vi "Trigger Controls with Data from CAT -sw1.vi"(5 "West ON/Std OFF":bool, 7 "Mode":enum16{"Run", "Hold", "Off"}(ring), 8 "error in":errorcluster, 11 "Com Parms":T2={"VISA resource name"="COM4", "baud rate"=38400, "data bits"=8, "parity"=0, "stop bits"=10, "flow control"=0} {"flow control" items=["None"=0, "XON/XOFF"=1, "RTS/CTS"=2, "DTR/DSR"=4]; "stop bits" items=["1.0"=10, "1.5"=15, "2.0"=20]; "parity" items=["None", "Odd", "Even", "Mark", "Space"]; "data bits" min=5 max=8 step=1}) -> (0 "error out":errorcluster, 3 "Final Output":T3={"Main 1"=TRUE, "Main 2"=TRUE, "Recirc  3"=TRUE, "Scrub 4"=FALSE, "O2 5"=TRUE, "Vent 6"=FALSE, "Boost A 7"=FALSE, "Boost A 8"=TRUE, "Recirc  9"=FALSE, "Scrub 10"=FALSE, "Vent 11"=FALSE, "Boost B 12"=TRUE, "Boost B 13"=TRUE, "Recirc 14"=TRUE, "Scrub 15"=FALSE, "Vent 16"=FALSE, "Main 17"=TRUE, "Boost A 18"=TRUE, "Boost B 19"=TRUE, "Boost F 20"=TRUE, "Vent 2 21"=FALSE})   [LabVIEW 2012]
uses:
  <vilib>/Platform/TimedLoop/XDataNode/XDataNode.xnode
  <vilib>/Platform/TimedLoop/XDataNode/nitl_modes.ctl
  <vilib>/Platform/TimedLoop/XDataNode/XDNodeRunTimeDep.lvlib
  <vilib>/Platform/TimedLoop/XDataNode/wakeup.ctl
  <vilib>/Platform/TimedLoop/XDataNode/timing_clust.ctl
  Type Defs/Final Output.ctl
  Type Defs/CO2 Settings.ctl
  Type Defs/AD Settings.ctl
  Type Defs/Output Values.ctl
  Type Defs/Output Switches.ctl
  Type Defs/Data Reading.ctl
panel:
  out "Time":string="16:44:30"
  out "Date":string="03/29/13"
  in  "Stop Button":bool
  in  "Tab Control":T1(tab)=enum."AD Settings"
  in  "Other Outputs":cluster{"Alarm":bool, "Heater":bool}
  in  "Period":i64=1000
  in  "Set Point Alt":dbl=1600.0 min=0.0 max=10000.0 step=1.0
  out "Cycles":i32=627
  out "CO2 ppm":u32(slide)=465 scale=0.0..10000.0
  out "Alt Dif M":dbl(slide)=-1619.283557610342 scale=-1000.0..1000.0 scale format="%.1f"
  out "AD Output":T3={"Main 1"=TRUE, "Main 2"=TRUE, "Recirc  3"=TRUE, "Scrub 4"=FALSE, "O2 5"=TRUE, "Vent 6"=FALSE, "Boost A 7"=FALSE, "Boost A 8"=TRUE, "Recirc  9"=FALSE, "Scrub 10"=FALSE, "Vent 11"=FALSE, "Boost B 12"=TRUE, "Boost B 13"=TRUE, "Recirc 14"=TRUE, "Scrub 15"=FALSE, "Vent 16"=FALSE, "Main 17"=TRUE, "Boost A 18"=TRUE, "Boost B 19"=TRUE, "Boost F 20"=TRUE, "Vent 2 21"=FALSE}
  out "AD State":T3
  out "Data Read":T4={"Date"="03/29/13", "Time"="16:44:31", "CO2- ppm"=467, "Last Ctrl Word"=5191831, "O2-1 ppm"=210267, "O2-2 ppm"=210262, "Temp MB"=23.23, "Temp Sensor Module"=26.21, "Press mB"=1011.26} {"Last Ctrl Word" format="%.0x"}
  out "Force Output":T5
  out "Force State":T3
  out "Alt Calc":dbl=-19.283557610342072
  in  "CO2 Settings":T6={"Run C1"={"A-1,  1"=inf, "A-3,  2"=inf, "A-4, 3"=9000.0, "A-5, 4"=8800.0, "ABCD-7, 5"=9600.0, "A-8, 6"=9200.0, "B-1,  7"=3400.0, "B-3, 8"=3400.0, "B-4,  9"=9000.0, "B-5, 10"=8800.0, "B-8, 11"=9200.0, "C-1, 12"=1800.0, "C-3, 13"=1800.0, "C-4, 14"=9000.0, "C-5,  15"=8800.0, "C-8, 16"=9200.0, "D-1, 17"=inf, "D-3, 18"=3400.0, "D-4,  19"=1800.0, "D-5,  20"=7000.0, "D-8,  21"=9200.0}, "Run C2"={"A-1,  1"=inf, "A-3,  2"=inf, "A-4, 3"=8800.0, "A-5, 4"=8600.0, "ABCD-7, 5"=9600.0, "A-8, 6"=9000.0, "B-1,  7"=3000.0, "B-3, 8"=3000.0, "B-4,  9"=8800.0, "B-5, 10"=8600.0, "B-8, 11"=9000.0, "C-1, 12"=1400.0, "C-3, 13"=1400.0, "C-4, 14"=8800.0, "C-5,  15"=8600.0, "C-8, 16"=9000.0, "D-1, 17"=inf, "D-3, 18"=3000.0, "D-4,  19"=1400.0, "D-5,  20"=6600.0, "D-8,  21"=9000.0}, "Hold C3"={"A-1,  1"=1800.0, "A-3,  2"=1800.0, "A-4, 3"=9000.0, "A-5, 4"=8800.0, "ABCD-7, 5"=9600.0, "A-8, 6"=9200.0, "B-1,  7"=3400.0, "B-3, 8"=3400.0, "B-4,  9"=9000.0, "B-5, 10"=8800.0, "B-8, 11"=9200.0, "C-1, 12"=1800.0, "C-3, 13"=1800.0, "C-4, 14"=9000.0, "C-5,  15"=8800.0, "C-8, 16"=9200.0, "D-1, 17"=1800.0, "D-3, 18"=3400.0, "D-4,  19"=1800.0, "D-5,  20"=7000.0, "D-8,  21"=9200.0}, "Hold C4"={"A-1,  1"=1400.0, "A-3,  2"=1400.0, "A-4, 3"=8800.0, "A-5, 4"=8600.0, "ABCD-7, 5"=9600.0, "A-8, 6"=9000.0, "B-1,  7"=3000.0, "B-3, 8"=3000.0, "B-4,  9"=8800.0, "B-5, 10"=8600.0, "B-8, 11"=9000.0, "C-1, 12"=1400.0, "C-3, 13"=1400.0, "C-4, 14"=8800.0, "C-5,  15"=8600.0, "C-8, 16"=9000.0, "D-1, 17"=1400.0, "D-3, 18"=3000.0, "D-4,  19"=1400.0, "D-5,  20"=6600.0, "D-8,  21"=9000.0}, "High CO2 Forces "={"A-1, 1"=TRUE, "A-3, 2"=TRUE, "A-4, 3"=FALSE, "A-5, 4"=TRUE, "ABCD-7, 5"=FALSE, "A-8, 6"=TRUE, "B-1,  7"=TRUE, "B-3, 8"=TRUE, "B-4, 9"=FALSE, "B-5, 10"=TRUE, "B-8,  11"=TRUE, "C-1, 12"=TRUE, "C-3, 13"=TRUE, "C-4,  14"=FALSE, "C-5,  15"=TRUE, "C-8, 16"=TRUE, "D-1, 17"=TRUE, "D-3, 18"=TRUE, "D-4, 19"=TRUE, "D-5,  20"=TRUE, "D-8,  21"=TRUE}}
  in  "AD Settings":T9={"Set Point Force"={"A-1,  1"=inf, "A-3,  2"=inf, "A-4, 3"=inf, "A-5, 4"=inf, "ABCD-7, 5"=inf, "A-8, 6"=inf, "B-1,  7"=inf, "B-3, 8"=inf, "B-4,  9"=inf, "B-5, 10"=inf, "B-8, 11"=inf, "C-1, 12"=inf, "C-3, 13"=inf, "C-4, 14"=inf, "C-5,  15"=inf, "C-8, 16"=inf, "D-1, 17"=inf, "D-3, 18"=inf, "D-4,  19"=inf, "D-5,  20"=6000.0, "D-8,  21"=inf}, "Run A1"={"A-1,  1"=inf, "A-3,  2"=inf, "A-4, 3"=50.0, "A-5, 4"=inf, "ABCD-7, 5"=50.0, "A-8, 6"=inf, "B-1,  7"=inf, "B-3, 8"=150.0, "B-4,  9"=60.0, "B-5, 10"=inf, "B-8, 11"=60.0, "C-1, 12"=15.0, "C-3, 13"=15.0, "C-4, 14"=50.0, "C-5,  15"=inf, "C-8, 16"=60.0, "D-1, 17"=inf, "D-3, 18"=0.0, "D-4,  19"=15.0, "D-5,  20"=0.0, "D-8,  21"=700.0}, "Run A2"={"A-1,  1"=inf, "A-3,  2"=inf, "A-4, 3"=-30.0, "A-5, 4"=inf, "ABCD-7, 5"=-30.0, "A-8, 6"=inf, "B-1,  7"=inf, "B-3, 8"=80.0, "B-4,  9"=15.0, "B-5, 10"=inf, "B-8, 11"=15.0, "C-1, 12"=-50.0, "C-3, 13"=-50.0, "C-4, 14"=-30.0, "C-5,  15"=inf, "C-8, 16"=15.0, "D-1, 17"=inf, "D-3, 18"=0.0, "D-4,  19"=-50.0, "D-5,  20"=-80.0, "D-8,  21"=650.0}, "Hold A3"={"A-1,  1"=0.0, "A-3,  2"=0.0, "A-4, 3"=50.0, "A-5, 4"=inf, "ABCD-7, 5"=50.0, "A-8, 6"=inf, "B-1,  7"=inf, "B-3, 8"=150.0, "B-4,  9"=60.0, "B-5, 10"=inf, "B-8, 11"=60.0, "C-1, 12"=-200.0, "C-3, 13"=-200.0, "C-4, 14"=50.0, "C-5,  15"=inf, "C-8, 16"=60.0, "D-1, 17"=0.0, "D-3, 18"=-150.0, "D-4,  19"=-200.0, "D-5,  20"=-200.0, "D-8,  21"=700.0}, "Hold A4"={"A-1,  1"=-150.0, "A-3,  2"=-150.0, "A-4, 3"=-30.0, "A-5, 4"=inf, "ABCD-7, 5"=-30.0, "A-8, 6"=inf, "B-1,  7"=inf, "B-3, 8"=80.0, "B-4,  9"=15.0, "B-5, 10"=inf, "B-8, 11"=15.0, "C-1, 12"=-300.0, "C-3, 13"=-300.0, "C-4, 14"=-30.0, "C-5,  15"=inf, "C-8, 16"=15.0, "D-1, 17"=-150.0, "D-3, 18"=-250.0, "D-4,  19"=-300.0, "D-5,  20"=-300.0, "D-8,  21"=650.0}, "High AD Diff "={"A-1, 1"=FALSE, "A-3, 2"=FALSE, "A-4, 3"=FALSE, "A-5, 4"=TRUE, "ABCD-7, 5"=FALSE, "A-8, 6"=TRUE, "B-1,  7"=TRUE, "B-3, 8"=FALSE, "B-4, 9"=TRUE, "B-5, 10"=TRUE, "B-8,  11"=TRUE, "C-1, 12"=FALSE, "C-3, 13"=FALSE, "C-4,  14"=FALSE, "C-5,  15"=TRUE, "C-8, 16"=TRUE, "D-1, 17"=FALSE, "D-3, 18"=FALSE, "D-4, 19"=FALSE, "D-5,  20"=FALSE, "D-8,  21"=TRUE}, "Delay S"={"A-1,  1"=30.0, "A-3,  2"=30.0, "A-4, 3"=1.0, "A-5, 4"=1.0, "ABCD-7, 5"=1.0, "A-8, 6"=1.0, "B-1,  7"=1.0, "B-3, 8"=1.0, "B-4,  9"=1.0, "B-5, 10"=1.0, "B-8, 11"=1.0, "C-1, 12"=30.0, "C-3, 13"=30.0, "C-4, 14"=1.0, "C-5,  15"=1.0, "C-8, 16"=1.0, "D-1, 17"=30.0, "D-3, 18"=30.0, "D-4,  19"=30.0, "D-5,  20"=30.0, "D-8,  21"=1.0}}
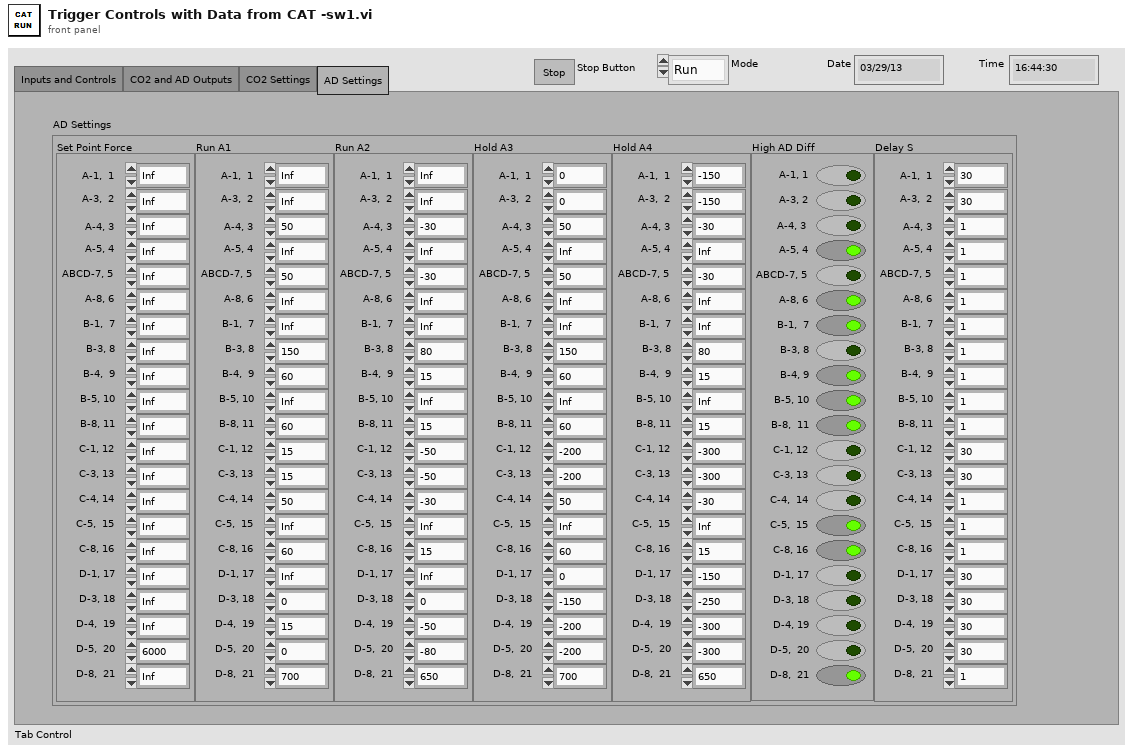
[diagram p1: front panel]
types:
  T1 = enum32{"Inputs and Controls", "CO2 and AD Outputs", "CO2 Settings", "AD Settings"}
  T2 = cluster{"VISA resource name":refnum<visa-resource-name>, "baud rate":u32, "data bits":u16, "parity":u16, "stop bits":u16, "flow control":u16}
  T3 = typedef "Final Output.ctl" = cluster{"Main 1":bool, "Main 2":bool, "Recirc  3":bool, "Scrub 4":bool, "O2 5":bool, "Vent 6":bool, "Boost A 7":bool, "Boost A 8":bool, "Recirc  9":bool, "Scrub 10":bool, "Vent 11":bool, "Boost B 12":bool, "Boost B 13":bool, "Recirc 14":bool, "Scrub 15":bool, "Vent 16":bool, "Main 17":bool, "Boost A 18":bool, "Boost B 19":bool, "Boost F 20":bool, "Vent 2 21":bool}
  T4 = typedef "Data Reading.ctl" = cluster{"Date":string, "Time":string, "CO2- ppm":u32, "Last Ctrl Word":u32, "O2-1 ppm":u32, "O2-2 ppm":u32, "Temp MB":sgl, "Temp Sensor Module":sgl, "Press mB":sgl}
  T5 = cluster{"Main 1":bool, "Main 2":bool, "Recirc  3":bool, "Scrub 4":bool, "O2 5":bool, "Vent 6":bool, "Boost A 7":bool, "Boost A 8":bool, "Recirc  9":bool, "Scrub 10":bool, "Vent 11":bool, "Boost B 12":bool, "Boost B 13":bool, "Recirc 14":bool, "Scrub 15":bool, "Vent 16":bool, "Main 17":bool, "Boost A 18":bool, "Boost B 19":bool, "Boost F 20":bool, "Vent 2 21":bool}
  T6 = typedef "CO2 Settings.ctl" = cluster{"Run C1":T7, "Run C2":T7, "Hold C3":T7, "Hold C4":T7, "High CO2 Forces ":T8}
  T7 = typedef "Output Values.ctl" = cluster{"A-1,  1":dbl, "A-3,  2":dbl, "A-4, 3":dbl, "A-5, 4":dbl, "ABCD-7, 5":dbl, "A-8, 6":dbl, "B-1,  7":dbl, "B-3, 8":dbl, "B-4,  9":dbl, "B-5, 10":dbl, "B-8, 11":dbl, "C-1, 12":dbl, "C-3, 13":dbl, "C-4, 14":dbl, "C-5,  15":dbl, "C-8, 16":dbl, "D-1, 17":dbl, "D-3, 18":dbl, "D-4,  19":dbl, "D-5,  20":dbl, "D-8,  21":dbl}
  T8 = typedef "Output Switches.ctl" = cluster{"A-1, 1":bool, "A-3, 2":bool, "A-4, 3":bool, "A-5, 4":bool, "ABCD-7, 5":bool, "A-8, 6":bool, "B-1,  7":bool, "B-3, 8":bool, "B-4, 9":bool, "B-5, 10":bool, "B-8,  11":bool, "C-1, 12":bool, "C-3, 13":bool, "C-4,  14":bool, "C-5,  15":bool, "C-8, 16":bool, "D-1, 17":bool, "D-3, 18":bool, "D-4, 19":bool, "D-5,  20":bool, "D-8,  21":bool}
  T9 = typedef "AD Settings.ctl" = cluster{"Set Point Force":T7, "Run A1":T7, "Run A2":T7, "Hold A3":T7, "Hold A4":T7, "High AD Diff ":T8, "Delay S":T7}
  T10 = cluster{"Date":string, "Time":string, "CO2- ppm":u32, "Last Ctrl Word":u32, "O2-1 ppm":u32, "O2-2 ppm":u32, "Temp MB":sgl, "Temp Sensor Module":sgl, "Press mB":sgl}
  T11 = cluster{"Main 1":bool, "Main 2":bool, "Recirc  3":bool, "Boost A 7":bool, "Recirc  9":bool, "Scrub 4":bool, "Scrub 10":bool, "O2 5":bool, "Vent 6":bool, "Boost A 8":bool, "Vent 11":bool, "Boost B 12":bool, "Boost B 13":bool, "Recirc 14":bool, "Scrub 15":bool, "Vent 16":bool, "Main 17":bool, "Boost A 18":bool, "Boost B 19":bool, "Boost F 20":bool, "Vent 2 21":bool}
  T12 = typedef "XDNodeRunTimeDep.lvlib/timing_clust.ctl" = cluster{"Expected End [f-1]":u64, "Actual End [f-1]":u64, "Finished Late? [f-1]":bool, "Expected End [i-1]":u64, "Actual End [i-1]":u64, "Finished Late? [i-1]":bool, "Expected Start [i]":u64, "Actual Start [i]":u64, "Expected Start [f]":u64, "Actual Start [f]":u64, "Source Name":string, "Structure Name":string, "Period":i64, "Deadline":i64, "Offset":i64, "Start":i64, "Priority":i32, "Timeout":i32, "Mode":T13, "Wakeup Reason":T14, "Error":errorcluster, "Source Type":string, "Secondary Source Type":string, "Global End Time":u64, "Global Start Time":u64, "Frame Duration":u64, "Iteration Duration":u64, "Assigned CPU":i32, "I/O Scan Engine Mode":u32}
  T13 = typedef "XDNodeRunTimeDep.lvlib/nitl_modes.ctl" = enum32{"No Change", "Process missed periods, maintain original phase", "Discard missed periods, maintain original phase", "Process missed periods, ignore original phase", "Discard missed periods, ignore original phase"}
  T14 = typedef "XDNodeRunTimeDep.lvlib/wakeup.ctl" = enum32{"Normal", "Aborted", "Asynchronous wakeup", "Timing source error", "Timed loop error", "Timeout"}
  T15 = cluster{"A-1,  1":bool, "A-3,  2":bool, "A-4, 3":bool, "A-5, 4":bool, "ABCD-7, 5":bool, "A-8, 6":bool, "B-1,  7":bool, "B-3, 8":bool, "B-4,  9":bool, "B-5, 10":bool, "B-8, 11":bool, "C-1, 12":bool, "C-3, 13":bool, "C-4, 14":bool, "C-5,  15":bool, "C-8, 16":bool, "D-1, 17":bool, "D-3, 18":bool, "D-4,  19":bool, "D-5,  20":bool, "D-8,  21":bool}
  T16 = cluster{bool, bool, bool, bool, bool, bool, bool, bool, bool, bool, bool, bool, bool, bool, bool, bool, bool, bool, bool, bool, bool}
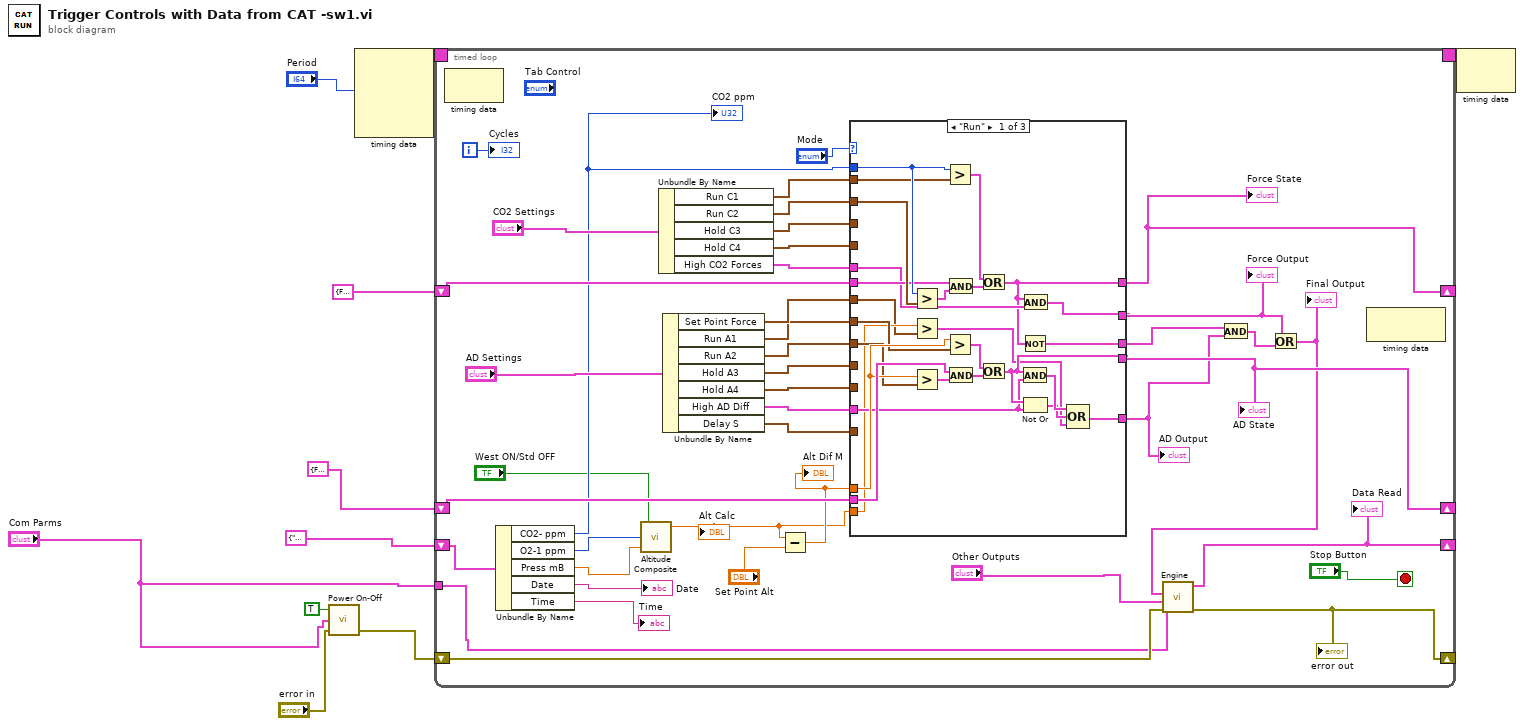
[diagram p0: block diagram]
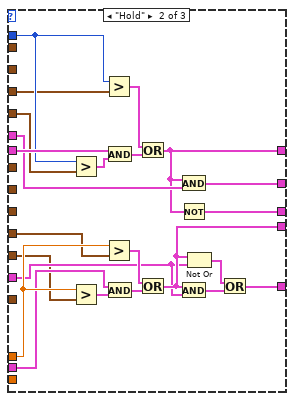
[diagram p2: hidden frame]
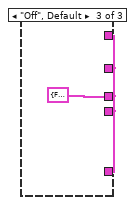
[diagram p3: hidden frame]
diagram:
  n1 = call "Power On-Off.vi"("error in"="error in", "Com Parms"="Com Parms", "On/Off"=TRUE) -> ("error out"=w3:errorcluster)  [unwired: 2 in]
  n2 = node-c288("Period") -> (w10:T12)  [unwired: 3 in]
  n3 = timed-loop {
    shift-right: [w51] -> _
    shift-left: T11 {"Main 1"=FALSE, "Main 2"=FALSE, "Recirc  3"=FALSE, "Boost A 7"=FALSE, "Recirc  9"=FALSE, "Scrub 4"=FALSE, "Scrub 10"=FALSE, "O2 5"=FALSE, "Vent 6"=FALSE, "Boost A 8"=FALSE, "Vent 11"=FALSE, "Boost B 12"=FALSE, "Boost B 13"=FALSE, "Recirc 14"=FALSE, "Scrub 15"=FALSE, "Vent 16"=FALSE, "Main 17"=FALSE, "Boost A 18"=FALSE, "Boost B 19"=FALSE, "Boost F 20"=FALSE, "Vent 2 21"=FALSE} -> [w50]
    shift-right: [w48] -> _
    shift-left: T11 {"Main 1"=FALSE, "Main 2"=FALSE, "Recirc  3"=FALSE, "Boost A 7"=FALSE, "Recirc  9"=FALSE, "Scrub 4"=FALSE, "Scrub 10"=FALSE, "O2 5"=FALSE, "Vent 6"=FALSE, "Boost A 8"=FALSE, "Vent 11"=FALSE, "Boost B 12"=FALSE, "Boost B 13"=FALSE, "Recirc 14"=FALSE, "Scrub 15"=FALSE, "Vent 16"=FALSE, "Main 17"=FALSE, "Boost A 18"=FALSE, "Boost B 19"=FALSE, "Boost F 20"=FALSE, "Vent 2 21"=FALSE} ("AD State") -> [w47]
    timing: w10 -> [_]
    timing-out: [_] -> w9
    shift-right: [w26] -> _
    shift-left: w3 -> [w27]
    tunnel: "Com Parms" -> [w14]
    shift-right: [w23] -> _
    shift-left: T10 {"Date"="", "Time"="", "CO2- ppm"=0, "Last Ctrl Word"=0, "O2-1 ppm"=0, "O2-2 ppm"=0, "Temp MB"=0.0, "Temp Sensor Module"=0.0, "Press mB"=0.0} ("Data Read") -> [w22]
    i -> [w49]
    stop <- "Stop Button" stop-if-true
    n4 = node-c288() -> ()  [unwired: 1 in, 1 out]
    n5 = Unbundle By Name(w22) -> ("CO2- ppm"=w21:u32, "O2-1 ppm"=w19:u32, "Press mB"=w18:sgl, "Date"=→"Date":string, "Time"=→"Time":string)
    "CO2 ppm" <- w21
    n6 = call "Altitude Composite.vi"("Pressure mBar"=w18, "O2ppm"=w19, "West ON/Std OFF"="West ON/Std OFF") -> ("Alt Eff M 1 correct"=w12:dbl)  [unwired: 2 out]
    "Alt Calc" <- w12
    n7 = Unbundle By Name("CO2 Settings") -> ("Run C1"=w28:T7, "Run C2"=w29:T7, "Hold C3"=w30:T7, "Hold C4"=w31:T7, "High CO2 Forces"=w32:T8)
    n8 = Unbundle By Name("AD Settings") -> ("Set Point Force"=w40:T7, "Run A1"=w39:T7, "Run A2"=w38:T7, "Hold A3"=w37:T7, "Hold A4"=w36:T7, "High AD Diff"=w35:T8, "Delay S"=w34:T7)
    n9 = Subtract(x=w12, y="Set Point Alt") -> (x-y=w17:dbl)
    "Alt Dif M" <- w17
    n10 = case shown="\"Run\"" "Mode" {
      tunnel: w21 -> [w78 w99 _]
      tunnel: w28 -> [w77 _ _]
      tunnel: [w55 w83 w103] -> w51
      tunnel: w29 -> [w79 _ _]
      tunnel: w30 -> [_ w98 _]
      tunnel: w31 -> [_ w97 _]
      tunnel: w50 -> [w74 w100 _]
      tunnel: w32 -> [w56 w89 _]
      tunnel: [w65 w90 w103] -> w46
      tunnel: w17 -> [w70 w94 _]
      tunnel: w39 -> [w69 _ _]
      tunnel: w38 -> [w68 _ _]
      tunnel: w37 -> [_ w81 _]
      tunnel: w36 -> [_ w80 _]
      tunnel: w34 -> [_ _ _]
      tunnel: w35 -> [w63 w87 _]
      tunnel: [w64 w88 w103] -> w48
      tunnel: w47 -> [w71 w93 _]
      tunnel: [w57 w84 w103] -> w45
      tunnel: w12 -> [w60 _ _]
      tunnel: w40 -> [w59 _ _]
      tunnel: [w54 w82 w103] -> w44
      frame "Run" {
        n11 = Greater?(x=w78, y=w79) -> (0:w67:T15)
        n12 = Greater?(x=w60, y=w59) -> (0:w58:T15)
        n13 = Greater?(x=w70, y=w68) -> (0:w66:T15)
        n14 = Greater?(x=w78, y=w77) -> (0:w76:T15)
        n15 = Greater?(x=w70, y=w69) -> (0:w73:T15)
        n16 = And(x=w74, y=w67) -> (x .and. y?=w75:T16)
        n17 = And(x=w71, y=w66) -> (x .and. y?=w72:T16)
        n18 = Or(x=w76, y=w75) -> (x .or. y?=w55:T16)
        n19 = Or(x=w73, y=w72) -> (x .or. y?=w64:T16)
        n20 = Not(x=w55) -> (.not. x?=w54:T16)
        n21 = And(x=w64, y=w63) -> (x .and. y?=w62:T8)
        n22 = Not Or(1:w63, 2:w64) -> (0:w61:T8)
        n23 = And(x=w55, y=w56) -> (x .and. y?=w65:T8)
        n24 = Compound Arithmetic op=OR(w62, w61, w58) -> (w57:T8)
      }
      frame "Hold" {
        n25 = Greater?(x=w99, y=w97) -> (0:w92:T15)
        n26 = Greater?(x=w94, y=w80) -> (0:w91:T15)
        n27 = Greater?(x=w99, y=w98) -> (0:w102:T15)
        n28 = Greater?(x=w94, y=w81) -> (0:w96:T15)
        n29 = And(x=w100, y=w92) -> (x .and. y?=w101:T16)
        n30 = And(x=w93, y=w91) -> (x .and. y?=w95:T16)
        n31 = Or(x=w102, y=w101) -> (x .or. y?=w83:T16)
        n32 = Or(x=w96, y=w95) -> (x .or. y?=w88:T16)
        n33 = And(x=w83, y=w89) -> (x .and. y?=w90:T8)
        n34 = Not(x=w83) -> (.not. x?=w82:T16)
        n35 = And(x=w88, y=w87) -> (x .and. y?=w85:T8)
        n36 = Not Or(1:w87, 2:w88) -> (0:w86:T8)
        n37 = Or(x=w86, y=w85) -> (x .or. y?=w84:T8)
      }
      frame "Off", Default {
        w103 = T11 {"Main 1"=FALSE, "Main 2"=FALSE, "Recirc  3"=FALSE, "Boost A 7"=FALSE, "Recirc  9"=FALSE, "Scrub 4"=FALSE, "Scrub 10"=FALSE, "O2 5"=FALSE, "Vent 6"=FALSE, "Boost A 8"=FALSE, "Vent 11"=FALSE, "Boost B 12"=FALSE, "Boost B 13"=FALSE, "Recirc 14"=FALSE, "Scrub 15"=FALSE, "Vent 16"=FALSE, "Main 17"=FALSE, "Boost A 18"=FALSE, "Boost B 19"=FALSE, "Boost F 20"=FALSE, "Vent 2 21"=FALSE}
      }
    }
    "Force State" <- w51
    "Force Output" <- w46
    "AD State" <- w48
    "AD Output" <- w45
    n38 = And(x=w44, y=w45) -> (x .and. y?=w43:T8)
    n39 = Or(x=w46, y=w43) -> (x .or. y?=w25:T8)
    "Final Output" <- w25
    n40 = call "Engine.vi"("error in"=w27, "Other Outputs"="Other Outputs", "Final Output Controls"=w25, "Com Parms"=w14) -> ("error out"=w26:errorcluster, "Data Read"=w23:T10)  [unwired: 3 in]
    "error out" <- w26
    "Data Read" <- w23
    n41 = node-c288() -> ()  [unwired: 1 in, 1 out]
    "Cycles" <- w49
  }
  n42 = node-c288(w9) -> ()  [unwired: 1 out]
